vi "Acquisition Message Loop.vi"(8 "error in (no error)":errorcluster, 9 "Data Queue":refnum<queue>, 10 "Data Notifier":refnum<notifier>, 11 "Message Queues":T1) -> (0 "error out":errorcluster)   [LabVIEW 2017, in "Acquisition.lvlib"]
doc: "Message loop for handling messages pertaining to the acquisition of data from the hardware."
uses:
  Acquisition.lvlib
  support/Message Queue/All Message Queues.ctl
  support/Message Queue/Message Cluster.ctl
  Hardware Configuration.ctl
  <vilib>/DAQmx/read.llb/DAQmx Read (Analog 1D Wfm NChan NSamp).vi
  support/Message Queue/Enqueue Message (Single).vi
  <vilib>/DAQmx/miscellaneous.llb/DAQmx Fill In Error Info.vi
  <vilib>/Utility/error.llb/Error Cluster From Error Code.vi
  <vilib>/ErrorRing/Error Ring.xnode
  support/Message Queue/Message Queue.lvlib
  <resource>/objmgr/daqmx.rc
panel:
  out "# waiting":i32
  out "# elements in queue":i32
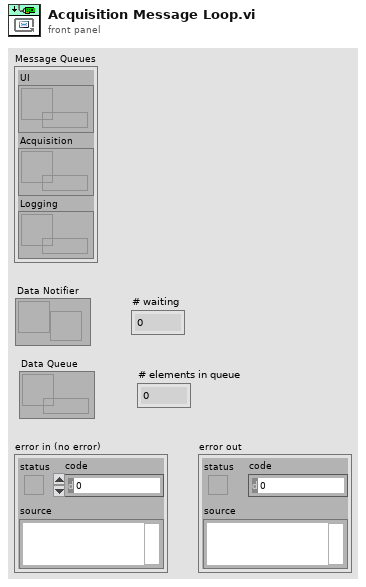
[diagram p1: front panel]
types:
  T1 = typedef "Message Queue.lvlib/All Message Queues.ctl" = cluster{"UI":refnum<queue>, "Acquisition":refnum<queue>, "Logging":refnum<queue>}
  T2 = typedef "Acquisition.lvlib/Hardware Configuration.ctl" = cluster{"DAQmx Input":tag, "Max Input":dbl, "Min Input":dbl, "Sample Rate":dbl, "DAQmx Task":refnum<k21>}
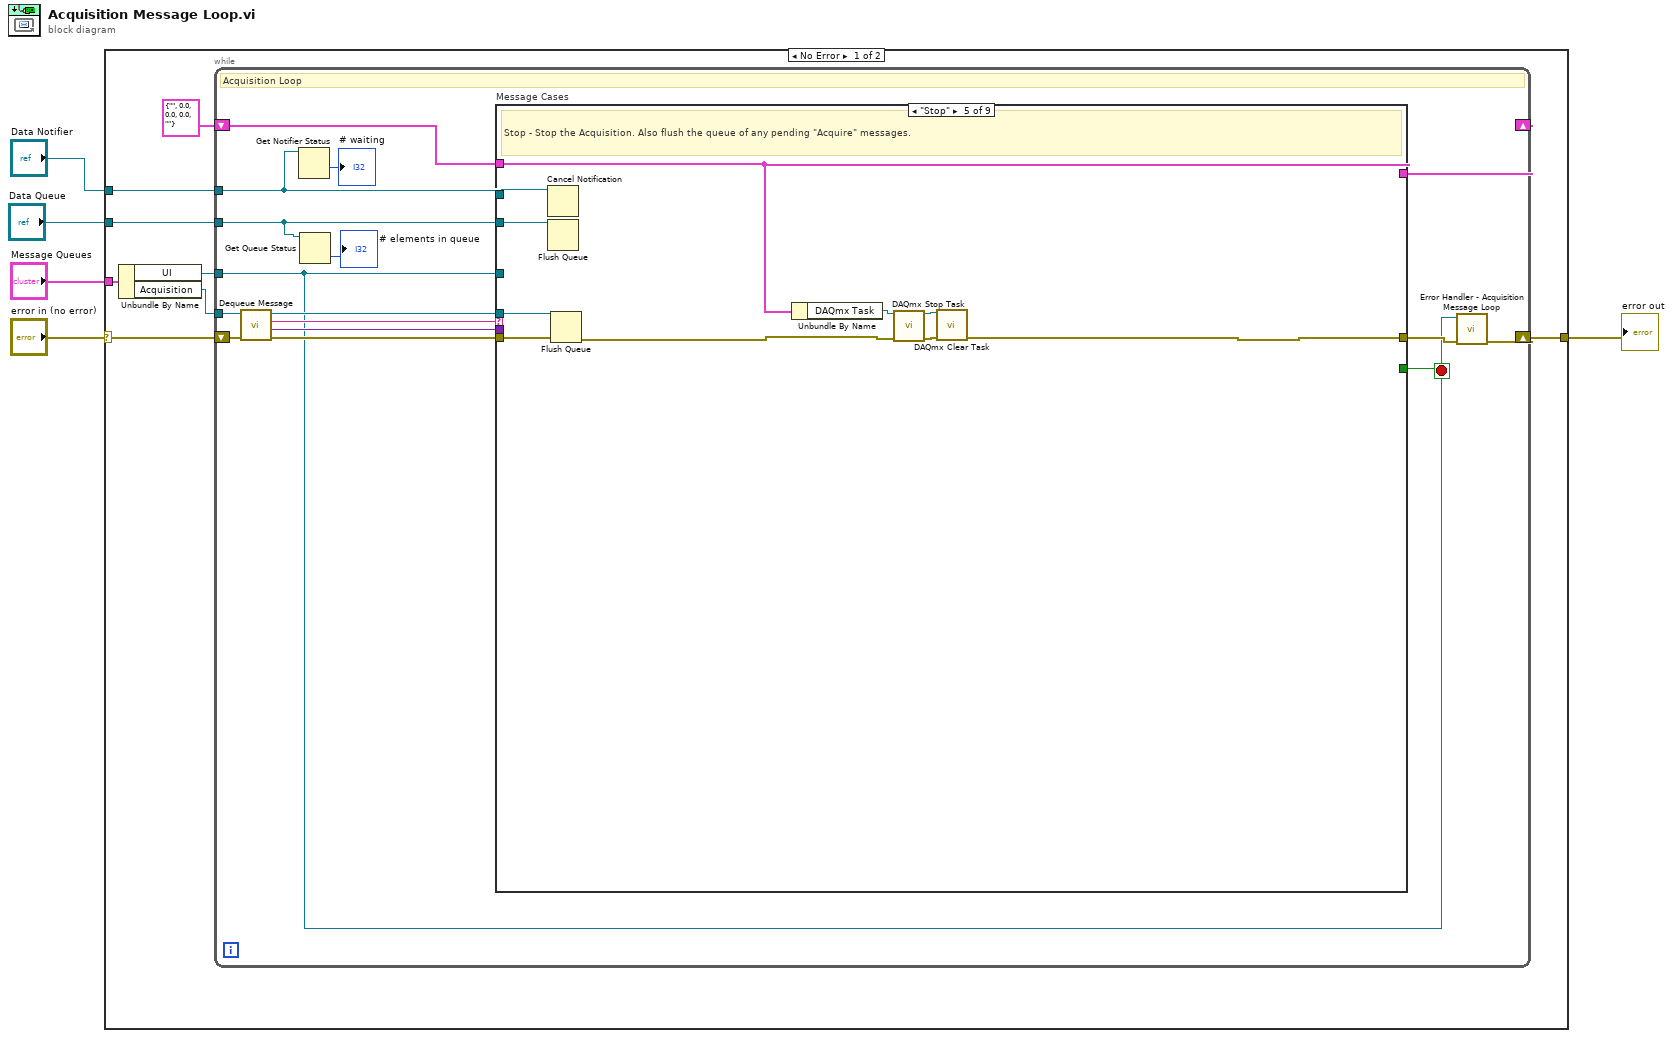
[diagram p0: block diagram]
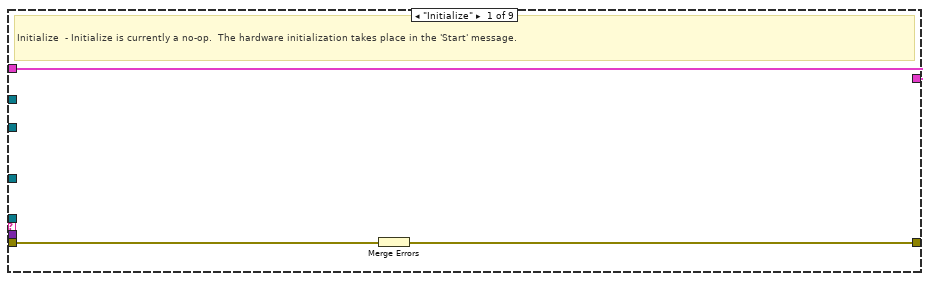
[diagram p2: hidden frame]
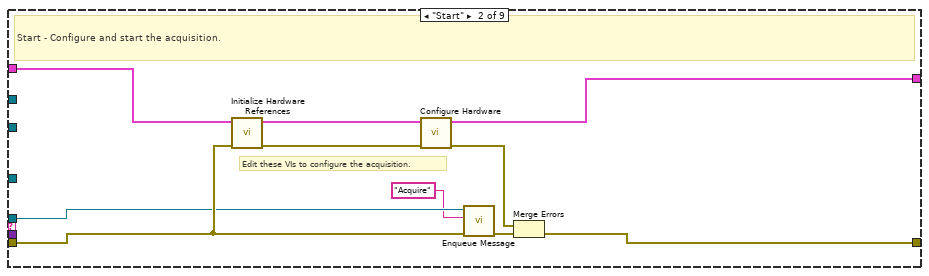
[diagram p3: hidden frame]
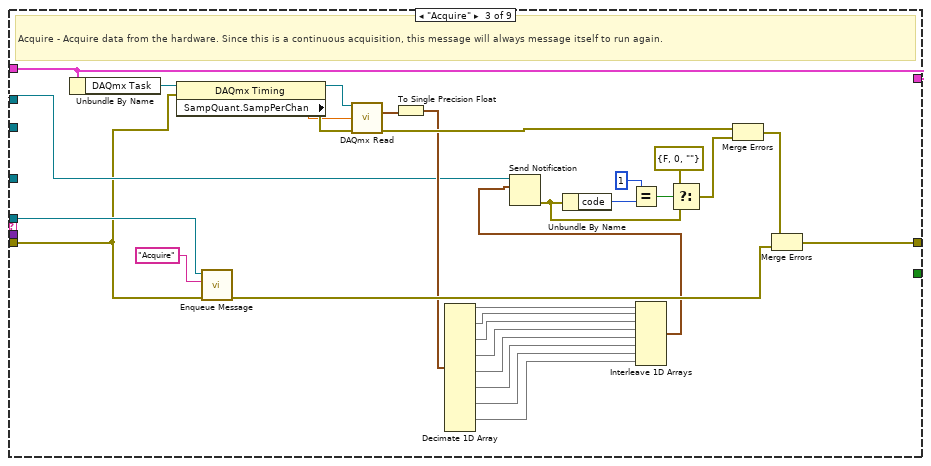
[diagram p4: hidden frame]
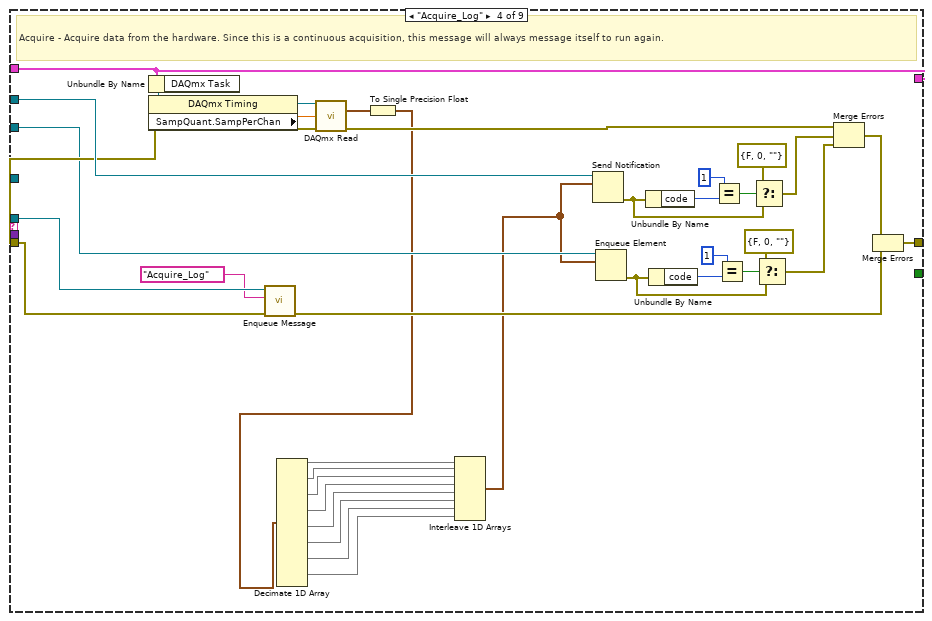
[diagram p5: hidden frame]
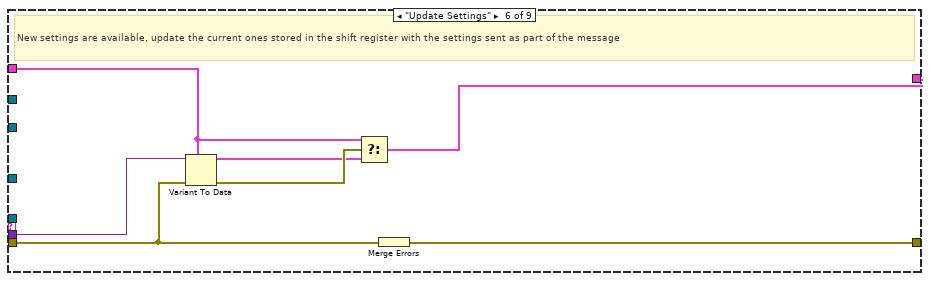
[diagram p6: hidden frame]
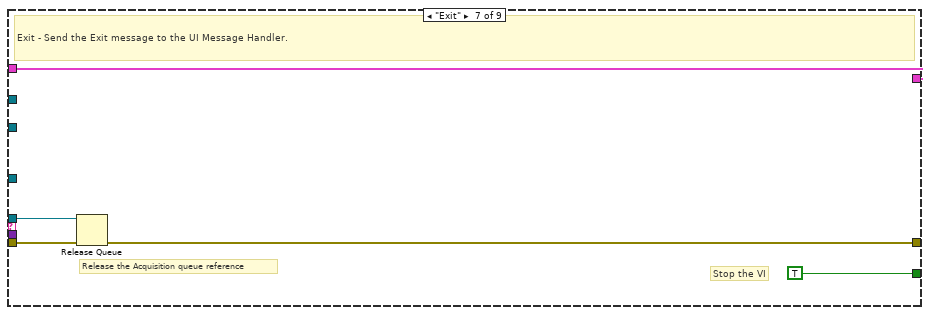
[diagram p7: hidden frame]
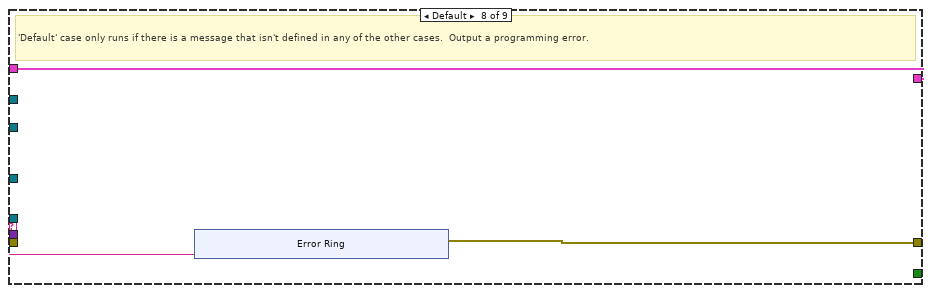
[diagram p8: hidden frame]
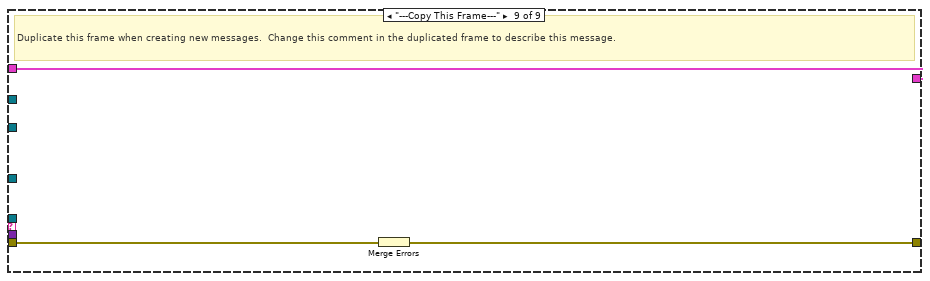
[diagram p9: hidden frame]
diagram:
  n1 = case shown="No Error" "error in (no error)" {
    selector: "error in (no error)" -> [w9 w145]
    tunnel: "Message Queues" -> [w13 _]
    tunnel: [w11 w145] -> w4
    tunnel: "Data Notifier" -> [w7 _]
    tunnel: "Data Queue" -> [w6 _]
    frame No Error {
      n2 = Unbundle By Name(w13) -> ("UI"=w8:refnum<queue>, "Acquisition"=w12:refnum<queue>)
      n3 = while {
        tunnel: w12 -> [w22]
        shift-right: [w18] -> _
        shift-left: T2 {"DAQmx Input"="", "Max Input"=0.0, "Min Input"=0.0, "Sample Rate"=0.0, "DAQmx Task"=""} ("Data Cluster") -> [w29]
        shift-right: [w20] -> w11
        shift-left: w9 -> [w27]
        tunnel: w8 -> [w19]
        tunnel: w7 -> [w16]
        tunnel: w6 -> [w14]
        stop <- w28 stop-if-true
        # "Acquisition Loop"
        n4 = call "Dequeue Message.vi"("error in (no error)"=w27, "Message Queue"=w22) -> ("error out"=w26:errorcluster, "Message Data"=w24:variant, "Message"=w25:string, "dup Message Queue"=w23:refnum<queue>)  [unwired: 6 in]
        n5 = Get Notifier Status(notifier=w16) -> (# waiting=→"# waiting":i32)  [unwired: 1 in, 4 out]
        n6 = Get Queue Status(queue=w14) -> (# elements in queue=→"# elements in queue":i32)  [unwired: 2 in, 7 out]
        n7 = case "Message Cases" shown="\"Stop\"" w25 {
          selector: w25 -> [_ _ _ _ _ _ _ w134 _]
          tunnel: w23 -> [_ w39 w70 w107 w118 _ w129 _ _]
          tunnel: w26 -> [w31 w40 w53 w86 w119 w121 w130 _ w144]
          tunnel: [w32 w42 w72 w109 w110 w126 w127 w133 w143] -> w21
          tunnel: w29 -> [w30 w41 w52 w85 w112 w122 w128 w132 w142]
          tunnel: [_ _ _ _ _ _ TRUE _ _] -> w28
          tunnel: w24 -> [_ _ _ _ _ w125 _ _ _]
          tunnel: w19 -> [_ _ _ _ _ _ _ _ _]
          tunnel: w16 -> [_ _ w54 w87 w117 _ _ _ _]
          tunnel: [w30 w38 w52 w85 w112 w120 w128 w132 w142] -> w18
          tunnel: w14 -> [_ _ _ w83 w111 _ _ _ _]
          frame "Initialize" {
            # "Initialize  - Initialize is currently a no-op.  The hardware initialization takes place in the 'Start' message."
            n8 = Merge Errors(w31) -> (w32:errorcluster)
          }
          frame "Start" {
            # "Edit these VIs to configure the acquisition."
            # "Start - Configure and start the acquisition."
            n9 = call "Initialize Hardware References.vi"("error in (no error)"=w40, "Hardware Resources in"=w41) -> ("error out"=w33:errorcluster, "Hardware Resources out"=w34:T2)  [unwired: 8 in]
            n10 = call "Configure Hardware.vi"("error in (no error)"=w33, "Hardware Resources in"=w34) -> ("error out"=w36:errorcluster, "Hardware Resources out"=w38:T2)  [unwired: 8 in]
            n11 = call-poly "Enqueue Message.vi"("error in (no error)"=w40, "Message"="Acquire", "Message Queue"=w39) -> ("error out"=w37:errorcluster)  [unwired: 7 in, 1 out]
            n12 = Merge Errors(w36, w37) -> (w42:errorcluster)
          }
          frame "Acquire" {
            # "Acquire - Acquire data from the hardware. Since this is a continuous acquisition, this message will always message itself to run again."
            n13 = Unbundle By Name(w52) -> ("DAQmx Task"=w60:refnum<k21>)
            n14 = property class="DAQmx Timing"(reference=w60, error in=w53) -> (reference out=w59:refnum<k21>, error out=w58:errorcluster, "SampQuant.SampPerChan"=w57:dbl)
            n15 = call-poly "Enqueue Message.vi"("error in (no error)"=w53, "Message"="Acquire", "Message Queue"=w70) -> ("error out"=w71:errorcluster)  [unwired: 7 in, 1 out]
            n16 = call-poly <vilib>:"DAQmx Read.vi"("task/channels in"=w59, "number of samples per channel"=w57, "error in"=w58) -> ("data"=w61:waveform(dbl)[], "error out"=w62:errorcluster)  [unwired: 10 in, 1 out]
            n17 = To Single Precision Float(number=w61) -> (single precision float=w56:waveform(sgl)[])
            n18 = Decimate 1D Array(w56) -> (w51:waveform(sgl)[], w50:waveform(sgl)[], w49:waveform(sgl)[], w48:waveform(sgl)[], w47:waveform(sgl)[], w46:waveform(sgl)[], w45:waveform(sgl)[], w44:waveform(sgl)[])  [unwired: 8 out]
            n19 = Interleave 1D Arrays(w51, w50, w49, w48, w47, w46, w45, w44) -> (w43:waveform(sgl)[])
            n20 = Send Notification(notification=w43, notifier=w54) -> (error out=w65:errorcluster)  [unwired: 1 in, 1 out]
            n21 = Unbundle By Name(w65) -> ("code"=w68:i32)
            n22 = Equal?(x=1, y=w68) -> (x = y?=w66:bool)
            n23 = Select(t=errorcluster {"status"=FALSE, "code"=0, "source"=""} ("error constant"), s=w66, f=w65) -> (s? t:f=w64:errorcluster)
            n24 = Merge Errors(w62, w64) -> (w55:errorcluster)
            n25 = Merge Errors(w55, w71) -> (w72:errorcluster)
          }
          frame "Acquire_Log" {
            # "Acquire - Acquire data from the hardware. Since this is a continuous acquisition, this message will always message itself to run again."
            n26 = Unbundle By Name(w85) -> ("DAQmx Task"=w92:refnum<k21>)
            n27 = property class="DAQmx Timing"(reference=w92, error in=w86) -> (reference out=w91:refnum<k21>, error out=w90:errorcluster, "SampQuant.SampPerChan"=w89:dbl)
            n28 = call-poly "Enqueue Message.vi"("error in (no error)"=w86, "Message"="Acquire_Log", "Message Queue"=w107) -> ("error out"=w108:errorcluster)  [unwired: 7 in, 1 out]
            n29 = call-poly <vilib>:"DAQmx Read.vi"("task/channels in"=w91, "number of samples per channel"=w89, "error in"=w90) -> ("data"=w84:waveform(dbl)[], "error out"=w93:errorcluster)  [unwired: 10 in, 1 out]
            n30 = To Single Precision Float(number=w84) -> (single precision float=w73:waveform(sgl)[])
            n31 = Decimate 1D Array(w73) -> (w82:waveform(sgl)[], w81:waveform(sgl)[], w80:waveform(sgl)[], w79:waveform(sgl)[], w78:waveform(sgl)[], w77:waveform(sgl)[], w76:waveform(sgl)[], w75:waveform(sgl)[])  [unwired: 8 out]
            n32 = Interleave 1D Arrays(w82, w81, w80, w79, w78, w77, w76, w75) -> (w74:waveform(sgl)[])
            n33 = Send Notification(notification=w74, notifier=w87) -> (error out=w102:errorcluster)  [unwired: 1 in, 1 out]
            n34 = Enqueue Element(queue=w83, element=w74) -> (error out=w98:errorcluster)  [unwired: 2 in, 2 out]
            n35 = Unbundle By Name(w102) -> ("code"=w105:i32)
            n36 = Unbundle By Name(w98) -> ("code"=w95:i32)
            n37 = Equal?(x=1, y=w105) -> (x = y?=w103:bool)
            n38 = Equal?(x=1, y=w95) -> (x = y?=w97:bool)
            n39 = Select(t=errorcluster {"status"=FALSE, "code"=0, "source"=""} ("error constant"), s=w103, f=w102) -> (s? t:f=w101:errorcluster)
            n40 = Select(t=errorcluster {"status"=FALSE, "code"=0, "source"=""} ("error constant"), s=w97, f=w98) -> (s? t:f=w94:errorcluster)
            n41 = Merge Errors(w93, w101, w94) -> (w88:errorcluster)
            n42 = Merge Errors(w88, w108) -> (w109:errorcluster)
          }
          frame "Stop" {
            # "Stop - Stop the Acquisition. Also flush the queue of any pending \"Acquire\" messages."
            n43 = Cancel Notification(0:w117) -> ()  [unwired: 1 in, 3 out]
            n44 = Flush Queue(queue=w111) -> ()  [unwired: 1 in, 3 out]
            n45 = Flush Queue(queue=w118, error in (no error)=w119) -> (error out=w113:errorcluster)  [unwired: 2 out]
            n46 = Unbundle By Name(w112) -> ("DAQmx Task"=w116:refnum<k21>)
            n47 = call <vilib>:"DAQmx Stop Task.vi"("task/channels in"=w116, "error in"=w113) -> ("task out"=w115:refnum<k21>, "error out"=w114:errorcluster)  [unwired: 12 in]
            n48 = call <vilib>:"DAQmx Clear Task.vi"("task in"=w115, "error in"=w114) -> ("error out"=w110:errorcluster)  [unwired: 13 in]
          }
          frame "Update Settings" {
            # "New settings are available, update the current ones stored in the shift register with the settings sent as part of the message"
            n49 = Variant To Data(error in=w121, type=w122, Variant=w125) -> (data=w123:T2, error out=w124:errorcluster)
            n50 = Select(t=w122, s=w124, f=w123) -> (s? t:f=w120:T2)
            n51 = Merge Errors(w121) -> (w126:errorcluster)
          }
          frame "Exit" {
            # "Release the Acquisition queue reference"
            # "Stop the VI"
            # "Exit - Send the Exit message to the UI Message Handler."
            n52 = Release Queue(queue=w129, error in (no error)=w130) -> (error out=w127:errorcluster)  [unwired: 1 in, 2 out]
          }
          frame Default {
            # "'Default' case only runs if there is a message that isn't defined in any of the other cases.  Output a programming error."
            n53 = xnode "Error Ring"("parameter 0"=w134) -> ("error out"=w133:errorcluster)
          }
          frame "---Copy This Frame---" {
            # "Duplicate this frame when creating new messages.  Change this comment in the duplicated frame to describe this message."
            n54 = Merge Errors(w144) -> (w143:errorcluster)
          }
        }
        n55 = call "Error Handler - Acquisition Message Loop.vi"("error in (no error)"=w21, "Message Queue"=w19) -> ("dup error in"=w20:errorcluster)  [unwired: 8 in, 1 out]
      }
    }
    frame Error {
    }
  }
  "error out" <- w4
